vi "SimEx Sine Test Labview Tutorial.vi"() -> ()   [LabVIEW 2020]
doc: "This example demonstrates how to generate a sine signal."
uses:
  <vilib>/Simulation/Scripting/Companion Diagram/SimConfigNode/SimParams.ctl
  <vilib>/Simulation/Scripting/Companion Diagram/SimConfigNode/_simSolvers.ctl
  <vilib>/Simulation/Implementation/Shared/SIMSCR Execution Mode.ctl
  <vilib>/Simulation/Param Hierarchy/ParamBlockSupport/SIMPH Read or Write Mode.ctl
  <vilib>/Platform/TimedLoop/XDataNode/timing_clust.ctl
  <vilib>/Platform/TimedLoop/XDataNode/nitl_modes.ctl
  <vilib>/Platform/TimedLoop/XDataNode/wakeup.ctl
  <vilib>/Simulation/Param Hierarchy/Typedefs/SIMPH Param Control Actions.ctl
  <vilib>/Simulation/Implementation/Shared/NILVSim_ParamChanged.vi
  <vilib>/Simulation/Implementation/Shared/NILVSim_FinishedLate.vi
  <vilib>/Simulation/Implementation/Shared/NILVSIM_BeginStep.vi
  <vilib>/Simulation/DataSources/Implementation/NILVSim Sine Wave.llb/SIM Sine Wave (scalar).vi
  <vilib>/Simulation/Utility/Implementation/SIM Halt.vi
  <vilib>/Simulation/Utility/Implementation/NILVSim Memory.llb/NILVSim Memory (core).vi
  <vilib>/Simulation/ContinuousLinear/Implementation/NILVSim Transfer Function.llb/SIM Transfer Function Distributor (SISO).vi
  <vilib>/Simulation/ContinuousLinear/Implementation/NILVSim Transfer Function.llb/SIM Transfer Function Collector (SISO).vi
  <vilib>/Simulation/ContinuousLinear/Implementation/NILVSim Zero Cross Detect.llb/SIM zero cross detect (scalar).vi
  <vilib>/Simulation/SignalDisplay/Implementation/NILVSim Time Waveform.llb/SIM Time Waveform (vector).vi
  <vilib>/Simulation/Implementation/Shared/NILVSim_Manager.vi
  <vilib>/Utility/error.llb/Clear Errors.vi
  <vilib>/Simulation/Implementation/Shared/NILVSim_FinalizeModel.vi
  <vilib>/Simulation/Implementation/Shared/SIM Unbundle Sim Info.vi
  <vilib>/Simulation/Implementation/Shared/SIMSH Read Queue.vi
  <vilib>/Simulation/Implementation/Shared/NILVSim_Initialize.vi
  <vilib>/Simulation/Utility/Implementation/NILVSim Get Time and IsAcceptedStep.vi
  <vilib>/Simulation/Implementation/Shared/NILVSim_GetModelError.vi
  <vilib>/Simulation/Implementation/Shared/SIM Bundle Sim Info.vi
  <vilib>/Simulation/Implementation/Shared/SIMSH Signal Block Listener.vi
  <vilib>/Simulation/Param Hierarchy/SIMPH Read Simulation Parameter.vi
  <vilib>/Simulation/Param Hierarchy/SIMPH Write Simulation Parameter.vi
  <vilib>/Simulation/Param Hierarchy/ParamBlockSupport/SIMPH Reset Call Chain.vi
  <vilib>/Simulation/Scripting/Companion Diagram/SimConfigNode/SimDog.xnode
  <vilib>/Platform/TimedLoop/XDataNode/XDataNode.xnode
  <vilib>/Simulation/Implementation/XNodeFramework/SimXNode/SimX.xnode
  <vilib>/Simulation/Param Hierarchy/ParamBlock/SIMPH_ParamBlock.xnode
  <vilib>/Simulation/ContinuousLinear/Implementation/NILVSim Transfer Function.llb/SIM Transfer Function (SISO).vi
  <vilib>/Platform/TimedLoop/XDataNode/XDNodeRunTimeDep.lvlib
  <vilib>/Simulation/Implementation/Shared/NI_SIM_Implementation.lvlib
panel:
  out "Waveform Chart 2":dbl[](graph)
  out "Gauge":dbl(knob) scale=-10.0..10.0
  in  "stop 2":bool
  out "Waveform Chart":waveform(dbl)[](graph)
  in  "stop":bool
  in  "Amplitude":dbl(slide)=1.0 scale=-5.0..5.0
  in  "Frequency (Hz)":dbl(slide)=0.5 scale=0.1..10.0
  in  "Phase":dbl(knob) scale=-275.0..275.0
  # "Overview: This example demonstrates how to generate a sine signal. Also show how to change parameters while the function is running.\nInstructions:\n1. Run the VI  and change the parameters of the sine signal on the front panel."
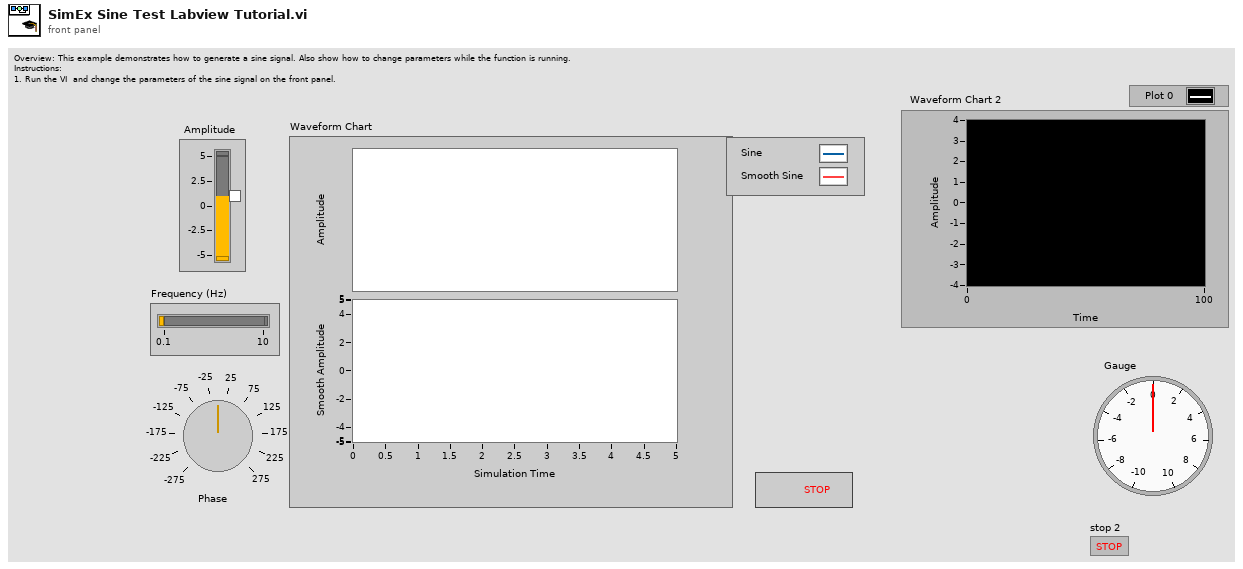
[diagram p1: front panel]
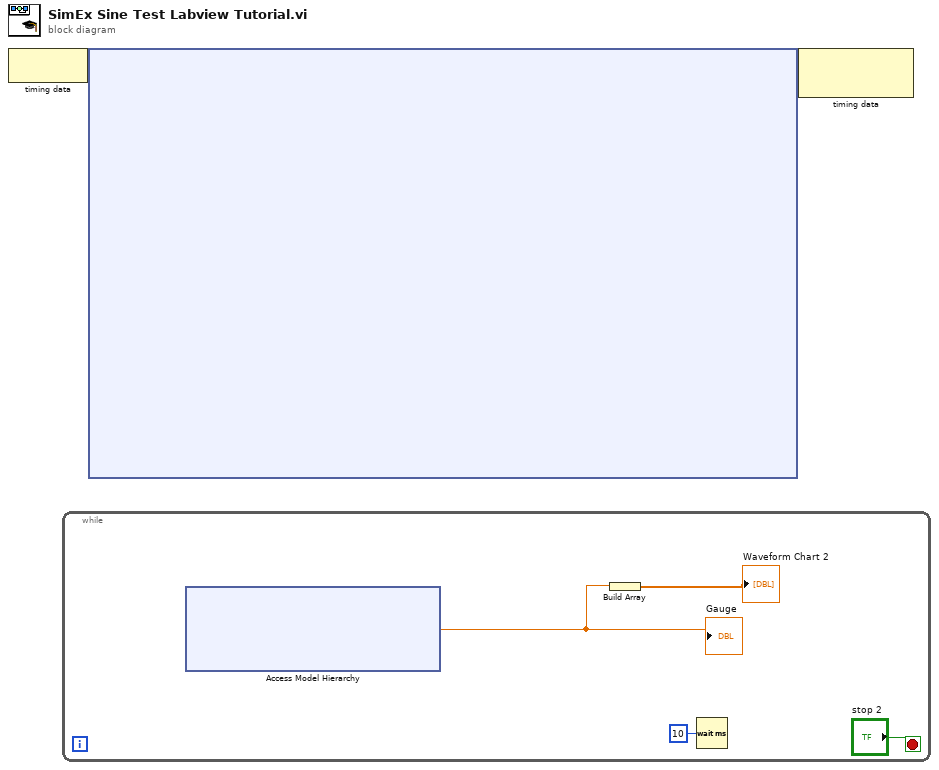
[diagram p0: block diagram]
diagram:
  n1 = node-c288() -> (w2:variant)  [unwired: 1 in]
  n2 = while {
    stop <- "stop 2" stop-if-true
    n3 = xnode ("Access Model Hierarchy")() -> ("Sine Signal.output"=w4:dbl)  [unwired: 2 in, 3 out]
    "Gauge" <- w4
    n4 = Build Array(w4) -> (→"Waveform Chart 2":dbl[])
    n5 = Wait (ms)(milliseconds to wait=u32 10) -> ()  [unwired: 1 out]
  }
  n6 = node-c254 ("Control & Simulation Loop")(w2) -> (w1:variant)
  n7 = node-c288(w1) -> ()  [unwired: 2 out]
